vi "Read Destroy.vi"(11 "Actor in":refnum<class "Actor.lvclass">) -> (2 "Destroy":bool)   [LabVIEW 2020, in "jettl.lvlib" / "Actor.lvlib" / "Actor.lvclass"]
uses:
  Actor.lvclass
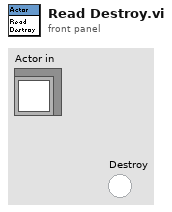
[diagram p1: front panel]
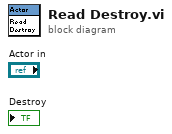
[diagram p0: block diagram]
diagram:
